vi "Tiempo_Prueba.vi"(8 "Error In":errorcluster) -> (0 "Error Out":errorcluster, 3 "current time":timestamp)   [LabVIEW 2013]
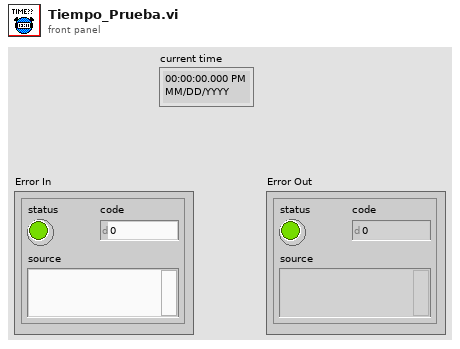
[diagram p1: front panel]
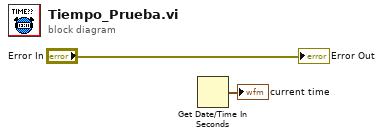
[diagram p0: block diagram]
diagram:
  n1 = Get Date/Time In Seconds() -> (seconds since 1Jan1904=→"current time":timestamp)
  "Error Out" <- "Error In"
